vi "Read_Excel_Document_to_Cluster_Array.vi"() -> (0 "SectionType_DATA":string[](array[string]), 1 "Cluster of 7 Type Data_5F":T2(array[cluster]), 2 "Cluster of 7 Type Data_DATA":T2(array[cluster]), 3 "Cluster of 7 Type Data_4F":T2(array[cluster]), 4 "Cluster of 7 Type Data_3F":T2(array[cluster]))   [LabVIEW 2014]
doc: "分别读取4楼、5楼和用于生成路径的数据"
uses:
  <vilib>/Analysis/Matrix/Datatypes/RealMatrix.ctl
  <vilib>/Analysis/Matrix/NI_Matrix.lvlib
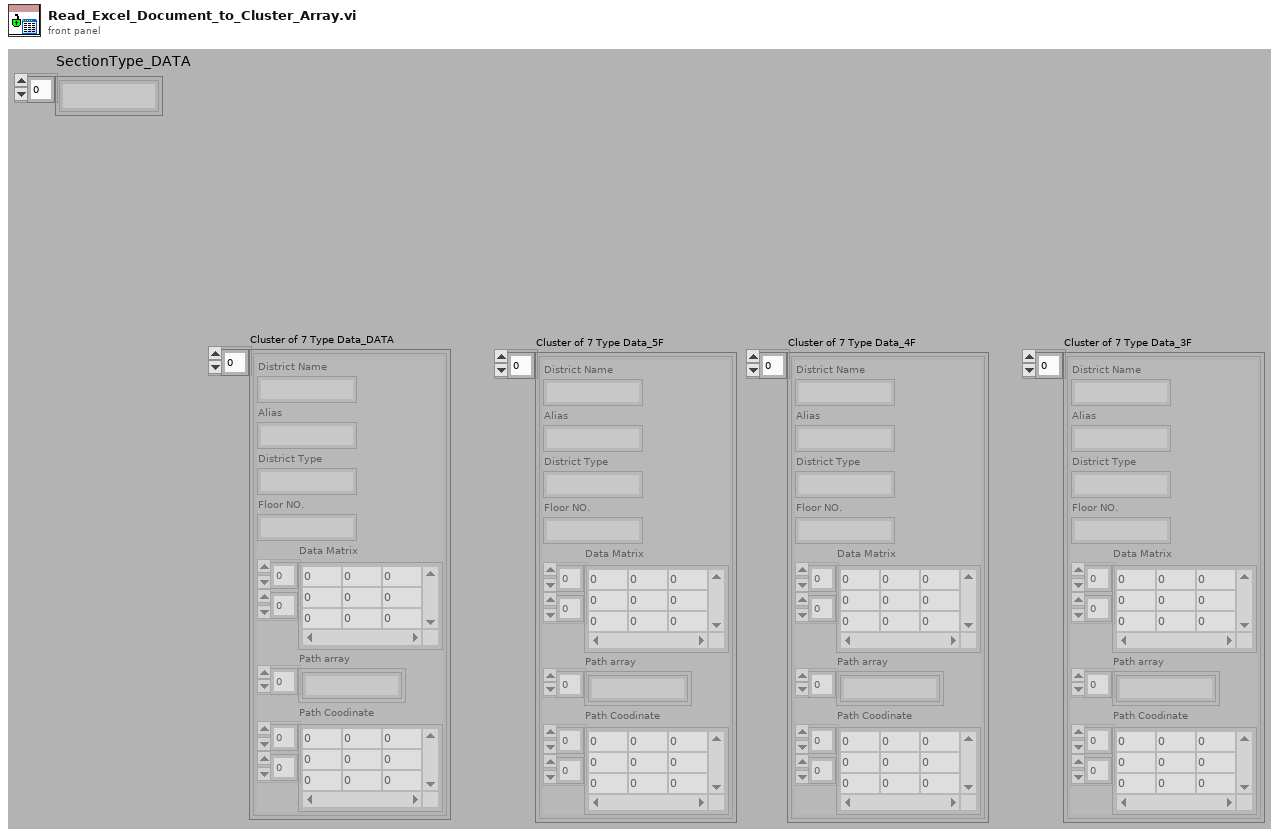
[diagram p1: front panel]
types:
  T1 = typedef "NI_Matrix.lvlib/RealMatrix.ctl" = dbl[][]
  T2 = cluster{"District Name":string, "Alias":string, "District Type":string, "Floor NO.":string, "Data Matrix":T1, "Path array":string[], "Path Coodinate":T1}[]
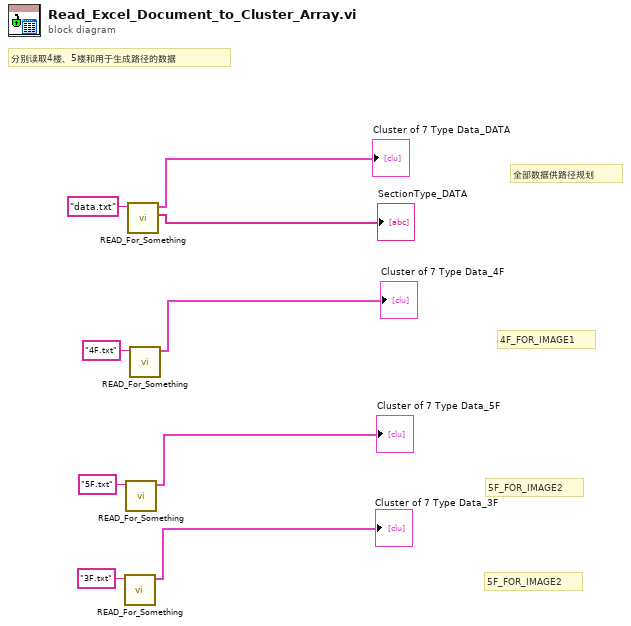
[diagram p0: block diagram]
diagram:
  # "5F_FOR_IMAGE2"
  # "分别读取4楼、5楼和用于生成路径的数据"
  # "5F_FOR_IMAGE2"
  # "4F_FOR_IMAGE1"
  # "全部数据供路径规划"
  n1 = call "READ_For_Something.vi"("名称"="3F.txt") -> ("数组 2"=→"Cluster of 7 Type Data_3F":T2)  [unwired: 9 in, 1 out]
  n2 = call "READ_For_Something.vi"("名称"="5F.txt") -> ("数组 2"=→"Cluster of 7 Type Data_5F":T2)  [unwired: 9 in, 1 out]
  n3 = call "READ_For_Something.vi"("名称"="data.txt") -> ("数组"=→"SectionType_DATA":string[], "数组 2"=→"Cluster of 7 Type Data_DATA":T2)  [unwired: 9 in]
  n4 = call "READ_For_Something.vi"("名称"="4F.txt") -> ("数组 2"=→"Cluster of 7 Type Data_4F":T2)  [unwired: 9 in, 1 out]
